vi "LVDimInterface.dis_set_quality.vi"(0 "my_serviceID":i32, 2 "quality":i32, 5 "error in (no error)":errorcluster) -> (14 "my_serviceID (out)":i32, 19 "error out":errorcluster)   [LabVIEW 2015, in "LVDimInterface.lvlib"]
doc: "Sets the quality of a DIM service\n\nHistory: 14-FEB-2006, Dietrich Beck\n\nCopyright (C)\nGesellschaft für Schwerionenforschung, GSI\nPlanckstr. 1\n64291 Darmstadt\nGermany\n\nContact: D.Beck@gsi.de \n\nThis program is free software; you can redistribute it and/or modify it under the terms of the \nGNU General Public License as published by the Free Software Foundation; either version 2 of the license, or (at your option) any later version.\n\nThis program is distributed in the hope that it will be useful, but WITHOUT ANY WARRANTY; without even the implied warranty of MERCHANTABILITY or FITNESS FOR A PARTICULAR PURPOSE. See the GNU General License for more details (http://www.gnu.org).\n\nGesellschaft für Schwerionenforschung, GSI\nPlanckstr. 1, 64291 Darmstadt, Germany\nFor all questions and ideas contact D. Beck.\nLast update: 16-DEC-2005"
uses:
  LVDimInterface.lvlib
  bin/libDimWrapper.dll
  bin/libDimWrapper.so
  bin/libDimWrapperSPL.dll
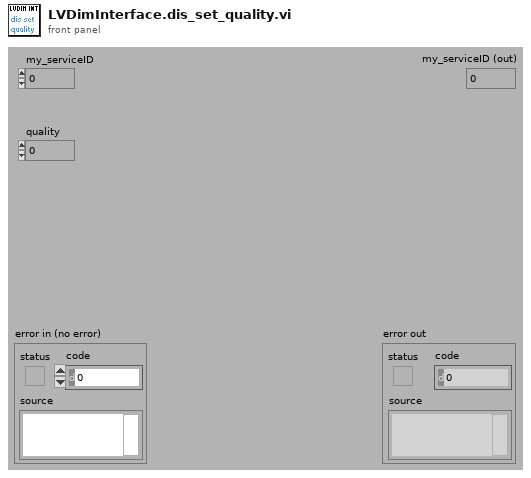
[diagram p1: front panel]
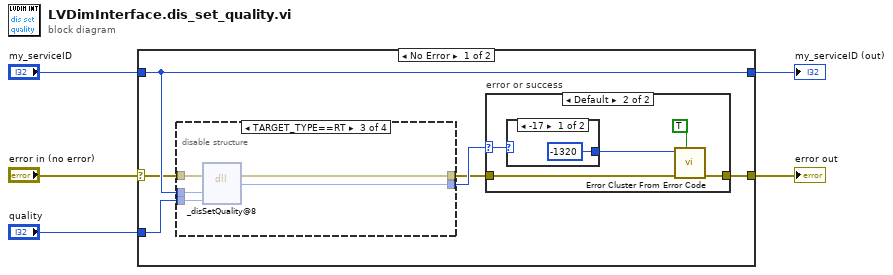
[diagram p0: block diagram]
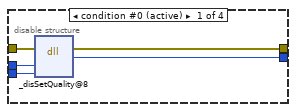
[diagram p2: hidden frame]
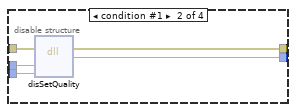
[diagram p3: hidden frame]
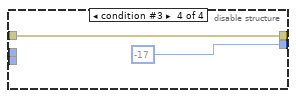
[diagram p4: hidden frame]
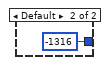
[diagram p6: hidden frame]
diagram:
  n1 = case shown="No Error" "error in (no error)" {
    selector: "error in (no error)" -> [w7 w37]
    tunnel: "my_serviceID" -> [w9 w38]
    tunnel: [w10 w37] -> w4
    tunnel: [w9 w38] -> w2
    tunnel: "quality" -> [w8 _]
    frame No Error {
      n2 = disable-structure "Conditional Disable Structure" shown="TARGET_TYPE==RT" {
        disable-tunnel: [w16 w21 w26 -17 ("error")] -> w11
        disable-tunnel: w9 -> [w15 w20 w25 _]
        disable-tunnel: w8 -> [w14 w19 w24 _]
        disable-tunnel: w7 -> [w13 w18 w23 w27]
        disable-tunnel: [w12 w17 w22 w27] -> w6
        frame condition #0 (active) {
          n3 = dll-call lib="D:/Git/CSPP/Packages/DimLVEvent/bin/libDimWrapper.dll" fn="_disSetQuality@8" label="disSetQuality"(error in=w13, "callBackID"=w15, "quality"=w14) -> (error out=w12:errorcluster, "error"=w16:i32)  [unwired: 4 in, 1 out]
        }
        frame condition #1 {
          n4 = dll-call lib="D:/Git/CS-framework/CSlibraries/DimLVEvent/bin/libDimWrapper.so" fn="disSetQuality"(error in=w18, "callBackID"=w20, "quality"=w19) -> (error out=w17:errorcluster, "error"=w21:i32)  [unwired: 4 in, 1 out]
        }
        frame condition #2 {
          n5 = dll-call lib="D:/Git/CS-framework/CSlibraries/DimLVEvent/bin/libDimWrapperSPL.dll" fn="_disSetQuality@8" label="libDimWrapper.so:disSetQuality"(error in=w23, "callBackID"=w25, "quality"=w24) -> (error out=w22:errorcluster, "error"=w26:i32)  [unwired: 4 in, 1 out]
        }
        frame condition #3 {
        }
      }
      n6 = case "error or success" shown="Default" w11 {
        selector: w11 -> [_ w34]
        tunnel: w6 -> [w29 w32]
        tunnel: [w29 w33] -> w10
        frame 0 {
        }
        frame Default {
          n7 = case shown="-17" w34 {
            tunnel: [-1320 ("code") -1316 ("code")] -> w31
            frame -17 {
            }
            frame Default {
            }
          }
          n8 = call <vilib>:"Error Cluster From Error Code.vi"("show call chain? (False)"=TRUE ("status"), "error in (no error)"=w32, "error code (0)"=w31) -> ("error out"=w33:errorcluster)  [unwired: 6 in]
        }
      }
    }
    frame Error {
    }
  }
  "error out" <- w4
  "my_serviceID (out)" <- w2
